vi "RSZVB Query Calibration Reference Plane Shift.vi"(8 "error in (no error)":errorcluster {"code" format="%.0x"}, 9 "Calibration Index (1)":i32=1, 10 "Channel (1)":i32=1, 11 "VISA session":refnum<visa-resource-name>) -> (0 "error out":errorcluster {"code" format="%.0x"}, 2 "Reference Plane Shift":dbl format="%^.3e", 3 "dup VISA session":refnum<visa-resource-name>)   [LabVIEW 2011]
doc: "This VI returns the reference plane shift to be applied to the result of a NIST Multiline TRL calibration. The <value> is entered as a mechanical length, where positive values denote a transformation towards the DUT, and negative values towards the connector.\n\nRemote-control command(s):\n[SENSe<Ch>:]CORRection:DATA:PARameter<Cal>? RPSHift"
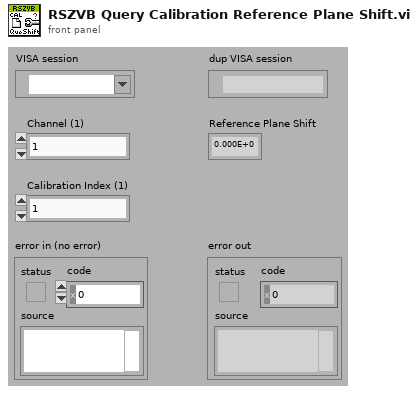
[diagram p1: front panel]
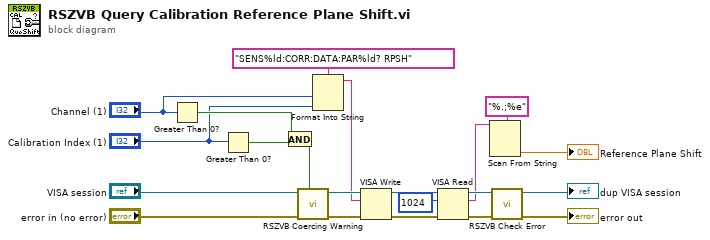
[diagram p0: block diagram]
diagram:
  n1 = Greater Than 0?(x="Channel (1)") -> (x > 0?=w6:bool)
  n2 = Greater Than 0?(x="Calibration Index (1)") -> (x > 0?=w7:bool)
  n3 = And(x=w6, y=w7) -> (x .and. y?=w5:bool)
  n4 = call "RSZVB Coercing Warning.vi"("In Range?"=w5, "error in (no error)"="error in (no error)", "VISA session"="VISA session") -> ("error out"=w19:errorcluster, "dup VISA session"=w20:refnum<visa-resource-name>)  [unwired: 7 in]
  n5 = Format Into String(format string="SENS%ld:CORR:DATA:PAR%ld? RPSH", "Channel (1)", "Calibration Index (1)") -> (resulting string=w18:string)  [unwired: 2 in, 1 out]
  n6 = VISA Write(VISA resource name=w20, write buffer=w18, error in (no error)=w19) -> (VISA resource name out=w11:refnum<visa-resource-name>, error out=w12:errorcluster)  [unwired: 1 out]
  n7 = VISA Read(VISA resource name=w11, byte count=u32 1024 ("byte count (0)"), error in (no error)=w12) -> (VISA resource name out=w16:refnum<visa-resource-name>, read buffer=w13:string, error out=w15:errorcluster)  [unwired: 1 out]
  n8 = Scan From String(format string="%.;%e", input string=w13) -> (output 1=→"Reference Plane Shift":dbl)  [unwired: 3 in, 3 out]
  n9 = call "RSZVB Check Error.vi"("error in (no error)"=w15, "VISA session"=w16) -> ("error out"=→"error out":errorcluster, "dup VISA session"=→"dup VISA session":refnum<visa-resource-name>)  [unwired: 8 in]
